vi "Stop Polling.vi"(8 "error in (no error)":errorcluster, 11 "Instruments in":refnum<class "Instruments.lvclass">) -> (0 "error out":errorcluster, 3 "Instruments out":refnum<class "Instruments.lvclass">)   [LabVIEW 2023, in "Instruments.lvlib" / "Instruments.lvclass"]
doc: "This stops the scheduled polling"
uses:
  Library/Instruments.lvclass
  Library/Instruments.lvclass/Instruments.ctl
  builds/Framework/Actor Framework.lvlibp/1abvi3w/vi.lib/ActorFramework/Time-Delayed Send Message/Time-Delay Override Options.ctl
  builds/Framework/Actor Framework.lvlibp
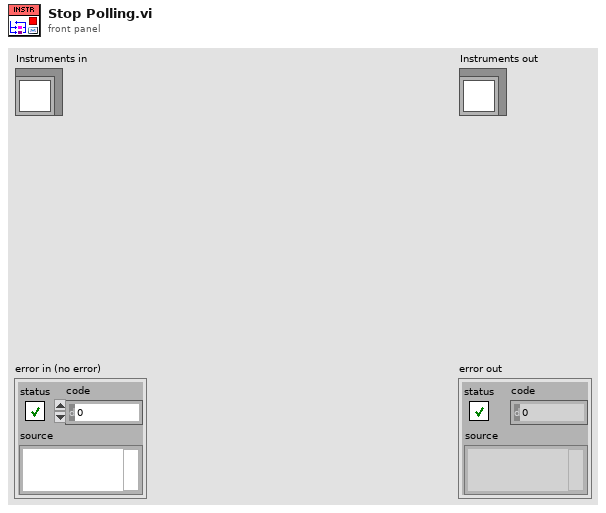
[diagram p1: front panel]
types:
  T1 = typedef "Actor Framework.lvlibp/Time-Delay Override Options.ctl" = enum16{"Send next copy now", "Skip next scheduled copy", "Send next copy now and stop all further copies", "Stop all further copies"}
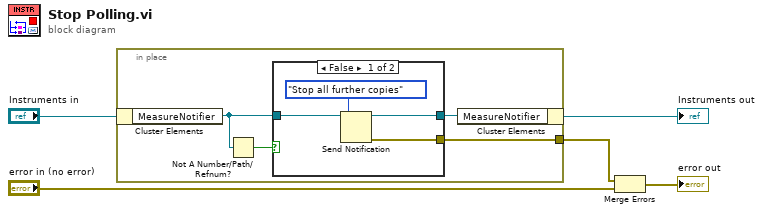
[diagram p0: block diagram]
diagram:
  n1 = in-place {
    in-place-border: [w8] -> w3
    n2 = in-place-cluster #1("Instruments in") -> ("MeasureNotifier"=w7:refnum<notifier>)
    n3 = Not A Number/Path/Refnum?(number/path/refnum=w7) -> (NaN/Path/Refnum?=w6:bool)
    n4 = case shown="False" w6 {
      tunnel: [w13 w14] -> w9
      tunnel: [w11 _] -> w8
      tunnel: w7 -> [w10 w14]
      frame False {
        n5 = Send Notification(notification=Time-Delay_Override_Options."Stop all further copies", notifier=w10) -> (notifier out=w13:refnum<notifier>, error out=w11:errorcluster)  [unwired: 1 in]
      }
      frame True {
      }
    }
    n6 = in-place-cluster #1("MeasureNotifier"=w9) -> (→"Instruments out":refnum<class "Instruments.lvclass">)
  }
  n7 = Merge Errors(w3, "error in (no error)") -> (→"error out":errorcluster)
